vi "WLAN Configure TxP.vi"(0 "Instrument Handle In":refnum<k21>, 1 "Selector String":string, 5 "TxP Configuration":T1={"Averaging Enabled"=0, "Averaging Count"=10, "Maximum Measurement Interval (s)"=0.001} {"Maximum Measurement Interval (s)" format="%.3p"; "Averaging Enabled" items=["False", "True"]}, 11 "error in (no error)":errorcluster) -> (4 "Instrument Handle Out":refnum<k21>, 15 "error out":errorcluster)   [LabVIEW 2016, in "RFmxWLAN.lvlib"]
doc: "Configures common settings for the TxP measurement and selects the measurement."
uses:
  RFmxWLAN.lvlib
  Typedefs/WLAN TxP Configuration.ctl
  <vilib>/RFmx/WLAN/mx/RFmxWLAN.llb/RFmxWLAN Select Measurement (Single).vi
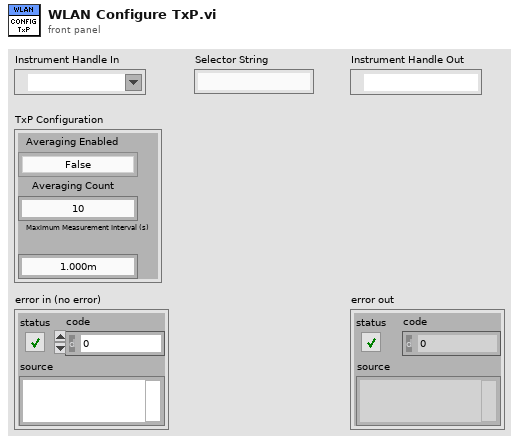
[diagram p1: front panel]
types:
  T1 = typedef "RFmxWLAN.lvlib/WLAN TxP Configuration.ctl" = cluster{"Averaging Enabled":i32, "Averaging Count":i32, "Maximum Measurement Interval (s)":dbl}
  T2 = enum16{"TXP", "PowerRamp", "DSSSModAcc", "OFDMModAcc", "SEM"}
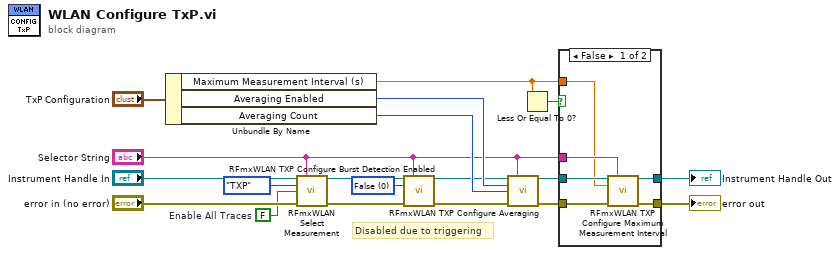
[diagram p0: block diagram]
diagram:
  w1 = FALSE  # Enable All Traces
  w5 = 0 items=["False", "True"] ("Burst Detection Enabled")
  # "Disabled due to triggering"
  n1 = Unbundle By Name("TxP Configuration") -> ("Maximum Measurement Interval (s)"=w9:dbl, "Averaging Enabled"=w11:i32, "Averaging Count"=w10:i32)
  n2 = call-poly <vilib>:"RFmxWLAN Select Measurement.vi"("Instrument Handle In"="Instrument Handle In", "Selector String"="Selector String", "Measurement"=T2."TXP", "Enable All Traces"=w1, "error in (no error)"="error in (no error)") -> ("Instrument Handle Out"=w7:refnum<k21>, "error out"=w17:errorcluster)  [unwired: 9 in]
  n3 = call <vilib>:"RFmxWLAN TXP Configure Burst Detection Enabled.vi"("Instrument Handle In"=w7, "Selector String"="Selector String", "Burst Detection Enabled"=w5, "error in (no error)"=w17) -> ("Instrument Handle Out"=w6:refnum<k21>, "error out"=w8:errorcluster)  [unwired: 10 in]
  n4 = call <vilib>:"RFmxWLAN TXP Configure Averaging.vi"("Instrument Handle In"=w6, "Selector String"="Selector String", "Averaging Enabled"=w11, "Averaging Count"=w10, "error in (no error)"=w8) -> ("Instrument Handle Out"=w13:refnum<k21>, "error out"=w14:errorcluster)  [unwired: 9 in]
  n5 = Less Or Equal To 0?(x=w9) -> (x <= 0?=w18:bool)
  n6 = case shown="False" w18 {
    tunnel: [w22 w27] -> w16
    tunnel: w13 -> [w23 w27]
    tunnel: [w24 w26] -> w15
    tunnel: w14 -> [w25 w26]
    tunnel: "Selector String" -> [w21 _]
    tunnel: w9 -> [w20 _]
    frame False {
      n7 = call <vilib>:"RFmxWLAN TXP Configure Maximum Measurement Interval.vi"("Instrument Handle In"=w23, "Selector String"=w21, "Maximum Measurement Interval (s)"=w20, "error in (no error)"=w25) -> ("Instrument Handle Out"=w22:refnum<k21>, "error out"=w24:errorcluster)  [unwired: 10 in]
    }
    frame True {
    }
  }
  "Instrument Handle Out" <- w16
  "error out" <- w15
